vi "CharacterizationDataReduction.vi"() -> ()   [LabVIEW 2018]
uses:
  <vilib>/Utility/file.llb/Read Delimited Spreadsheet (DBL).vi
panel:
  out "XY Graph":cluster{"all rows":dbl[], "all rows":dbl[]}(graph)
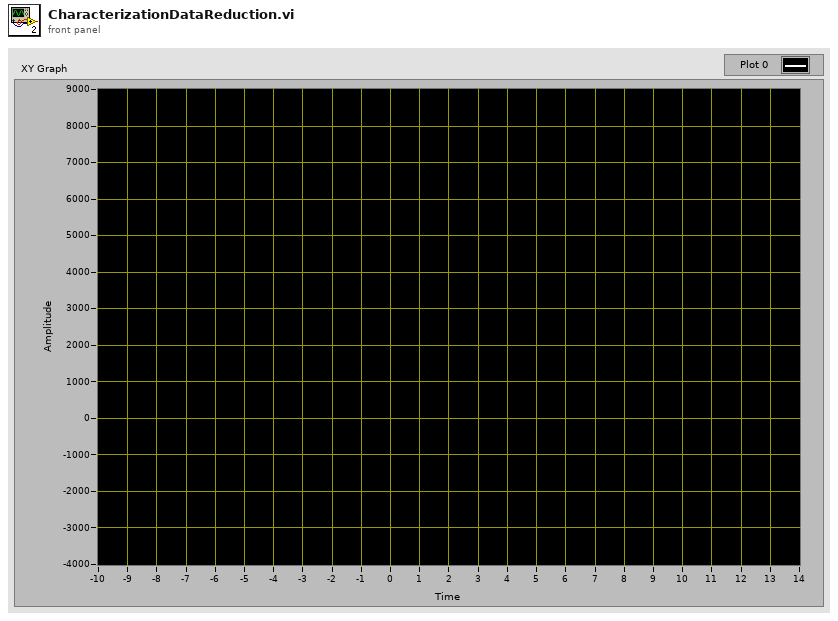
[diagram p1: front panel]
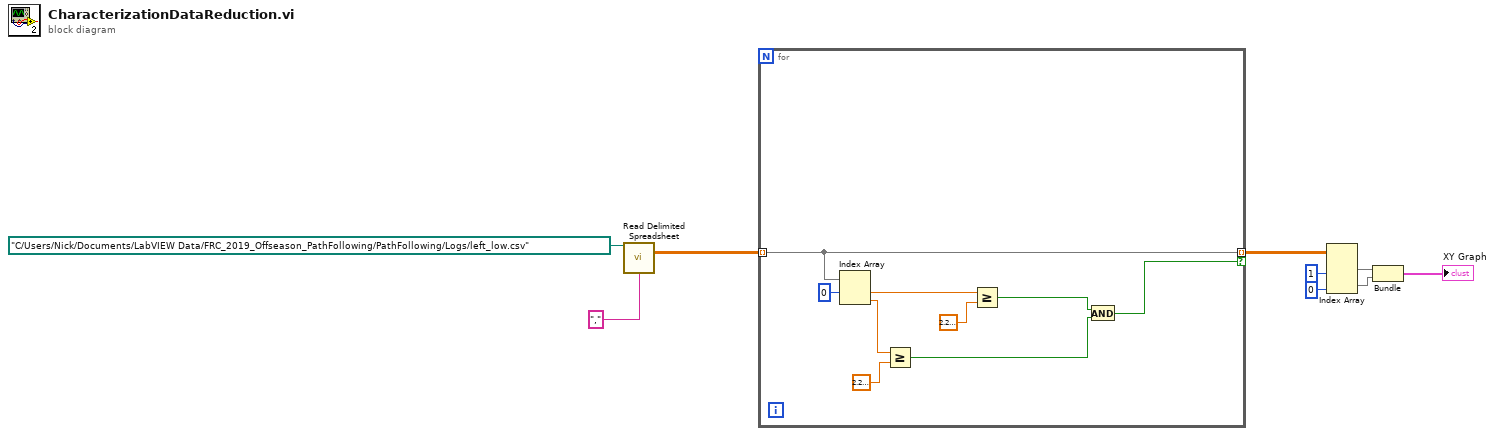
[diagram p0: block diagram]
diagram:
  n1 = call-poly <vilib>:"Read Delimited Spreadsheet.vi"("file path (dialog if empty)"=path "C:/Users/Nick/Documents/LabVIEW Data/FRC_2019_Offseason_PathFollowing/PathFollowing/Logs/left_low.csv", "delimiter (\\t)"="," ("delimiter (\\t)")) -> ("all rows"=w7:dbl[][])  [unwired: 8 in, 5 out]
  n2 = for {
    tunnel: w7 -> [w18] mode=indexing
    tunnel: [w18] -> w6 mode=indexing if=w10
    n3 = Index Array(array=w18, index #1=0 ("index")) -> (element #1=w16:dbl, element #2=w13:dbl)  [unwired: 1 in]
    n4 = Greater Or Equal?(x=w13, y=2.220446049250313e-16) -> (x >= y?=w12:bool)
    n5 = Greater Or Equal?(x=w16, y=2.220446049250313e-16) -> (x >= y?=w11:bool)
    n6 = And(x=w11, y=w12) -> (x .and. y?=w10:bool)
  }
  n7 = Index Array(array=w6, index (col) #1=1 ("disabled index (col)"), index (col) #2=0 ("index (col)")) -> (element #1=w3:dbl[], element #2=w2:dbl[])  [unwired: 2 in]
  n8 = Bundle("all rows"=w3, "all rows"=w2) -> (→"XY Graph":cluster{"all rows":dbl[], "all rows":dbl[]})  [unwired: 1 in]
